vi "device_init_all_FISH02.vi"() -> ()   [LabVIEW 2019]
uses:
  device/TETECH_TC720.llb/TC720.lvclass
  device/SV_LG16ch.llb/SV_LG16ch.lvclass
  device/CAVRO_XC.llb/XC3P.lvclass
  device/VICI EMHCA.llb/VICI EMHCA_10PORTS.lvclass
  device/device_global.vi
panel:
  in  "SV_LG16ch.lvclass":refnum<class "SV_LG16ch.lvclass">
  in  "TC720 in":refnum<class "TC720.lvclass">
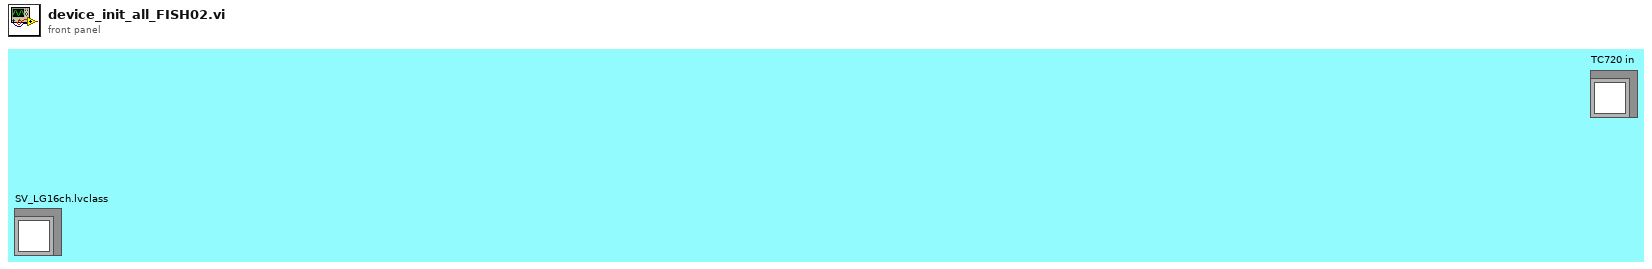
[diagram p1: front panel]
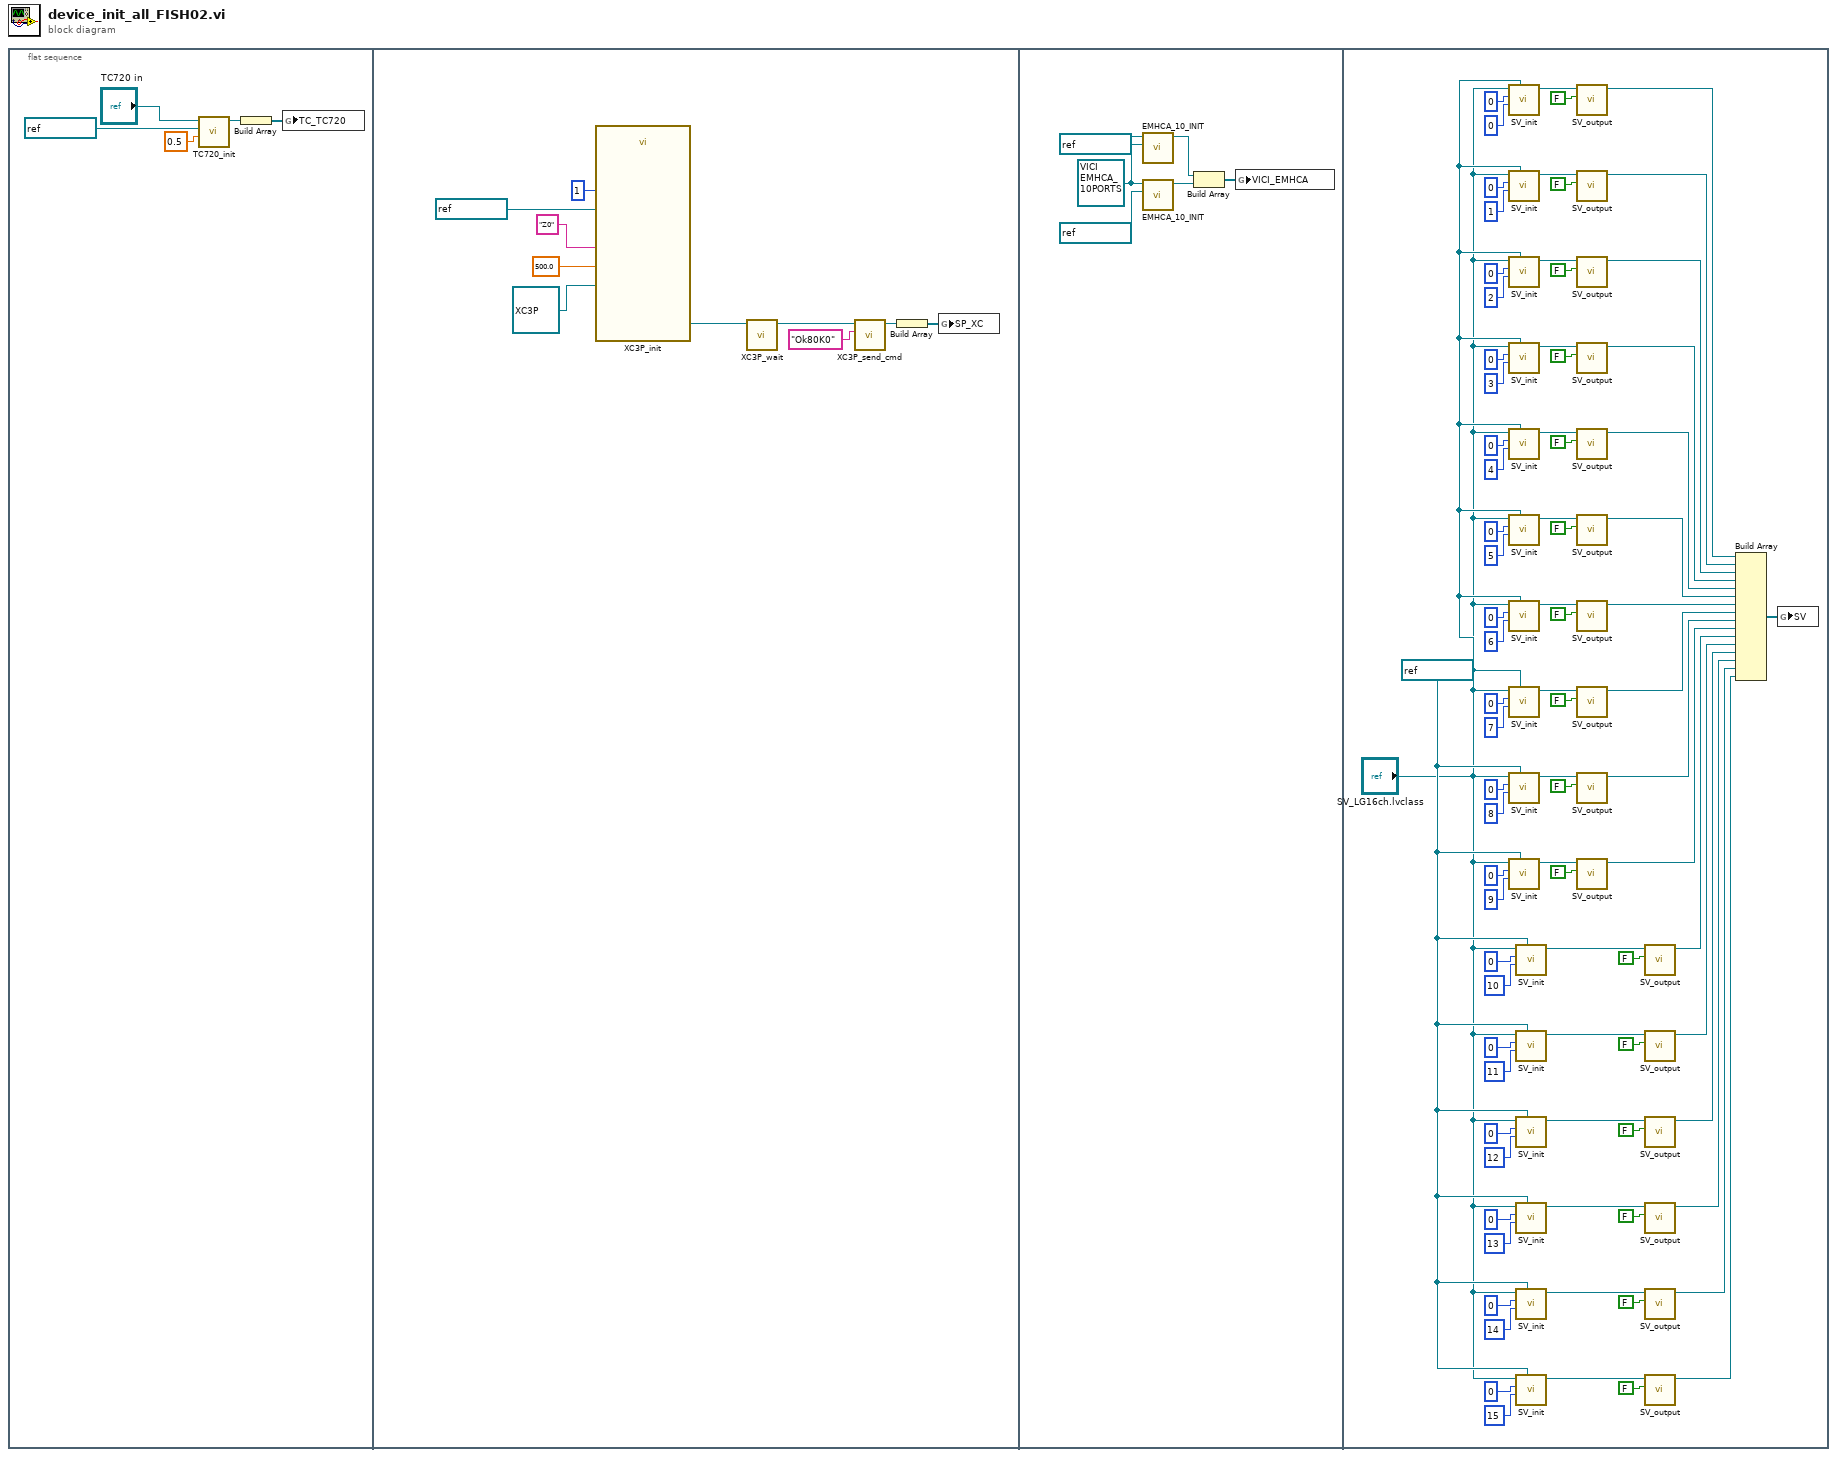
[diagram p0: block diagram]
diagram:
  n1 = flat-sequence {
    frame #0 {
      n2 = call-dynamic "TC720_init.vi"("temp_ready_dead_zone"=0.5, "COM PORT"=refnum<visa-resource-name> "COM15", "TC720 in"="TC720 in") -> ("TC720 out"=w3:refnum<class "TC720.lvclass">)  [unwired: 7 in, 1 out]
      n3 = Build Array(w3) -> (w2:refnum<class "TC720.lvclass">[])
      n4 = global write "device_global.vi" "TC_TC720"(w2) -> ()
    }
    frame #1 {
      n5 = call-dynamic "XC3P_init.vi"("address"=u8 1, "COM PORT"=refnum<visa-resource-name> "COM19", "syringe_volumn"=500.0, "mode"="Z0", "XC3P in"=refnum<class "XC3P.lvclass"> refnum ("XC3P.lvclass")) -> ("XC3P out"=w9:refnum<class "XC3P.lvclass">)  [unwired: 5 in, 1 out]
      n6 = call-dynamic "XC3P_wait.vi"("XC3P in"=w9) -> ("XC3P out"=w11:refnum<class "XC3P.lvclass">)  [unwired: 8 in, 2 out]
      n7 = call-dynamic "XC3P_send_cmd.vi"("Command"="Ok80K0", "XC3P in"=w11) -> ("XC3P out"=w6:refnum<class "XC3P.lvclass">)  [unwired: 6 in, 3 out]
      n8 = Build Array(w6) -> (w7:refnum<class "XC3P.lvclass">[])
      n9 = global write "device_global.vi" "SP_XC"(w7) -> ()
    }
    frame #2 {
      w18 = refnum<class "VICI EMHCA_10PORTS.lvclass"> refnum ("VICI EMHCA_10PORTS.lvclass")
      n10 = call-dynamic "EMHCA_10_INIT.vi"("COM PORT"=refnum<visa-resource-name> "COM17", "VICI EMHCA_10PORTS in"=w18) -> ("VICI EMHCA_10PORTS out"=w20:refnum<class "VICI EMHCA_10PORTS.lvclass">)  [unwired: 8 in, 1 out]
      n11 = call-dynamic "EMHCA_10_INIT.vi"("COM PORT"=refnum<visa-resource-name> "COM18", "VICI EMHCA_10PORTS in"=w18) -> ("VICI EMHCA_10PORTS out"=w16:refnum<class "VICI EMHCA_10PORTS.lvclass">)  [unwired: 8 in, 1 out]
      n12 = Build Array(w20, w16) -> (w19:refnum<class "VICI EMHCA_10PORTS.lvclass">[])
      n13 = global write "device_global.vi" "VICI_EMHCA"(w19) -> ()
    }
    frame #3 {
      w23 = refnum<visa-resource-name> "COM16" ("COM PORT")
      n14 = call-dynamic "SV_init.vi"("COM PORT"=w23, "Port Address"=u8 0, "Board Address"=u8 0, "SV_LG16ch in"="SV_LG16ch.lvclass") -> ("SV_LG16ch out"=w34:refnum<class "SV_LG16ch.lvclass">)  [unwired: 6 in, 1 out]
      n15 = call-dynamic "SV_init.vi"("COM PORT"=w23, "Port Address"=u8 1, "Board Address"=u8 0, "SV_LG16ch in"="SV_LG16ch.lvclass") -> ("SV_LG16ch out"=w32:refnum<class "SV_LG16ch.lvclass">)  [unwired: 6 in, 1 out]
      n16 = call-dynamic "SV_init.vi"("COM PORT"=w23, "Port Address"=u8 2, "Board Address"=u8 0, "SV_LG16ch in"="SV_LG16ch.lvclass") -> ("SV_LG16ch out"=w30:refnum<class "SV_LG16ch.lvclass">)  [unwired: 6 in, 1 out]
      n17 = call-dynamic "SV_init.vi"("COM PORT"=w23, "Port Address"=u8 3, "Board Address"=u8 0, "SV_LG16ch in"="SV_LG16ch.lvclass") -> ("SV_LG16ch out"=w67:refnum<class "SV_LG16ch.lvclass">)  [unwired: 6 in, 1 out]
      n18 = call-dynamic "SV_init.vi"("COM PORT"=w23, "Port Address"=u8 4, "Board Address"=u8 0, "SV_LG16ch in"="SV_LG16ch.lvclass") -> ("SV_LG16ch out"=w76:refnum<class "SV_LG16ch.lvclass">)  [unwired: 6 in, 1 out]
      n19 = call-dynamic "SV_init.vi"("COM PORT"=w23, "Port Address"=u8 5, "Board Address"=u8 0, "SV_LG16ch in"="SV_LG16ch.lvclass") -> ("SV_LG16ch out"=w79:refnum<class "SV_LG16ch.lvclass">)  [unwired: 6 in, 1 out]
      n20 = call-dynamic "SV_init.vi"("COM PORT"=w23, "Port Address"=u8 6, "Board Address"=u8 0, "SV_LG16ch in"="SV_LG16ch.lvclass") -> ("SV_LG16ch out"=w84:refnum<class "SV_LG16ch.lvclass">)  [unwired: 6 in, 1 out]
      n21 = call-dynamic "SV_init.vi"("COM PORT"=w23, "Port Address"=u8 7, "Board Address"=u8 0, "SV_LG16ch in"="SV_LG16ch.lvclass") -> ("SV_LG16ch out"=w92:refnum<class "SV_LG16ch.lvclass">)  [unwired: 6 in, 1 out]
      n22 = call-dynamic "SV_init.vi"("COM PORT"=w23, "Port Address"=u8 8, "Board Address"=u8 0, "SV_LG16ch in"="SV_LG16ch.lvclass") -> ("SV_LG16ch out"=w93:refnum<class "SV_LG16ch.lvclass">)  [unwired: 6 in, 1 out]
      n23 = call-dynamic "SV_init.vi"("COM PORT"=w23, "Port Address"=u8 9, "Board Address"=u8 0, "SV_LG16ch in"="SV_LG16ch.lvclass") -> ("SV_LG16ch out"=w100:refnum<class "SV_LG16ch.lvclass">)  [unwired: 6 in, 1 out]
      n24 = call-dynamic "SV_init.vi"("COM PORT"=w23, "Port Address"=u8 10, "Board Address"=u8 0, "SV_LG16ch in"="SV_LG16ch.lvclass") -> ("SV_LG16ch out"=w60:refnum<class "SV_LG16ch.lvclass">)  [unwired: 6 in, 1 out]
      n25 = call-dynamic "SV_init.vi"("COM PORT"=w23, "Port Address"=u8 11, "Board Address"=u8 0, "SV_LG16ch in"="SV_LG16ch.lvclass") -> ("SV_LG16ch out"=w53:refnum<class "SV_LG16ch.lvclass">)  [unwired: 6 in, 1 out]
      n26 = call-dynamic "SV_init.vi"("COM PORT"=w23, "Port Address"=u8 12, "Board Address"=u8 0, "SV_LG16ch in"="SV_LG16ch.lvclass") -> ("SV_LG16ch out"=w52:refnum<class "SV_LG16ch.lvclass">)  [unwired: 6 in, 1 out]
      n27 = call-dynamic "SV_init.vi"("COM PORT"=w23, "Port Address"=u8 13, "Board Address"=u8 0, "SV_LG16ch in"="SV_LG16ch.lvclass") -> ("SV_LG16ch out"=w45:refnum<class "SV_LG16ch.lvclass">)  [unwired: 6 in, 1 out]
      n28 = call-dynamic "SV_init.vi"("COM PORT"=w23, "Port Address"=u8 14, "Board Address"=u8 0, "SV_LG16ch in"="SV_LG16ch.lvclass") -> ("SV_LG16ch out"=w44:refnum<class "SV_LG16ch.lvclass">)  [unwired: 6 in, 1 out]
      n29 = call-dynamic "SV_init.vi"("COM PORT"=w23, "Port Address"=u8 15, "Board Address"=u8 0, "SV_LG16ch in"="SV_LG16ch.lvclass") -> ("SV_LG16ch out"=w25:refnum<class "SV_LG16ch.lvclass">)  [unwired: 6 in, 1 out]
      n30 = call-dynamic "SV_output.vi"("OUTPUT"=FALSE, "SV_LG16ch in"=w34) -> ("SV_LG16ch out"=w33:refnum<class "SV_LG16ch.lvclass">)  [unwired: 8 in, 1 out]
      n31 = call-dynamic "SV_output.vi"("OUTPUT"=FALSE, "SV_LG16ch in"=w32) -> ("SV_LG16ch out"=w31:refnum<class "SV_LG16ch.lvclass">)  [unwired: 8 in, 1 out]
      n32 = call-dynamic "SV_output.vi"("OUTPUT"=FALSE, "SV_LG16ch in"=w30) -> ("SV_LG16ch out"=w29:refnum<class "SV_LG16ch.lvclass">)  [unwired: 8 in, 1 out]
      n33 = call-dynamic "SV_output.vi"("OUTPUT"=FALSE, "SV_LG16ch in"=w67) -> ("SV_LG16ch out"=w94:refnum<class "SV_LG16ch.lvclass">)  [unwired: 8 in, 1 out]
      n34 = call-dynamic "SV_output.vi"("OUTPUT"=FALSE, "SV_LG16ch in"=w76) -> ("SV_LG16ch out"=w95:refnum<class "SV_LG16ch.lvclass">)  [unwired: 8 in, 1 out]
      n35 = call-dynamic "SV_output.vi"("OUTPUT"=FALSE, "SV_LG16ch in"=w79) -> ("SV_LG16ch out"=w96:refnum<class "SV_LG16ch.lvclass">)  [unwired: 8 in, 1 out]
      n36 = call-dynamic "SV_output.vi"("OUTPUT"=FALSE, "SV_LG16ch in"=w84) -> ("SV_LG16ch out"=w97:refnum<class "SV_LG16ch.lvclass">)  [unwired: 8 in, 1 out]
      n37 = call-dynamic "SV_output.vi"("OUTPUT"=FALSE, "SV_LG16ch in"=w92) -> ("SV_LG16ch out"=w98:refnum<class "SV_LG16ch.lvclass">)  [unwired: 8 in, 1 out]
      n38 = call-dynamic "SV_output.vi"("OUTPUT"=FALSE, "SV_LG16ch in"=w93) -> ("SV_LG16ch out"=w99:refnum<class "SV_LG16ch.lvclass">)  [unwired: 8 in, 1 out]
      n39 = call-dynamic "SV_output.vi"("OUTPUT"=FALSE, "SV_LG16ch in"=w100) -> ("SV_LG16ch out"=w104:refnum<class "SV_LG16ch.lvclass">)  [unwired: 8 in, 1 out]
      n40 = call-dynamic "SV_output.vi"("OUTPUT"=FALSE, "SV_LG16ch in"=w60) -> ("SV_LG16ch out"=w40:refnum<class "SV_LG16ch.lvclass">)  [unwired: 8 in, 1 out]
      n41 = call-dynamic "SV_output.vi"("OUTPUT"=FALSE, "SV_LG16ch in"=w53) -> ("SV_LG16ch out"=w39:refnum<class "SV_LG16ch.lvclass">)  [unwired: 8 in, 1 out]
      n42 = call-dynamic "SV_output.vi"("OUTPUT"=FALSE, "SV_LG16ch in"=w52) -> ("SV_LG16ch out"=w38:refnum<class "SV_LG16ch.lvclass">)  [unwired: 8 in, 1 out]
      n43 = call-dynamic "SV_output.vi"("OUTPUT"=FALSE, "SV_LG16ch in"=w45) -> ("SV_LG16ch out"=w37:refnum<class "SV_LG16ch.lvclass">)  [unwired: 8 in, 1 out]
      n44 = call-dynamic "SV_output.vi"("OUTPUT"=FALSE, "SV_LG16ch in"=w44) -> ("SV_LG16ch out"=w36:refnum<class "SV_LG16ch.lvclass">)  [unwired: 8 in, 1 out]
      n45 = call-dynamic "SV_output.vi"("OUTPUT"=FALSE, "SV_LG16ch in"=w25) -> ("SV_LG16ch out"=w24:refnum<class "SV_LG16ch.lvclass">)  [unwired: 8 in, 1 out]
      n46 = Build Array(w33, w31, w29, w94, w95, w96, w97, w98, w99, w104, w40, w39, w38, w37, w36, w24) -> (w35:refnum<class "SV_LG16ch.lvclass">[])
      n47 = global write "device_global.vi" "SV"(w35) -> ()
    }
  }
